vi "Redis@PreviewQueue__Parameter.vi"(1 "ParamterIn":string) -> (0 "ParamterOut":string)   [LabVIEW 2020]
panel:
  in  "Message=":string
  in  "TimeOut=":string(combo)
  in  "Variable=":string(combo)
  in  "Section":string(combo)
  in  "CMD":string
  in  "RedisSession":string(combo)
  in  "Confirm":bool
  # "RedisSession(,Variable=,TimeOut=XXX, Message=XXX)"
  # "@"
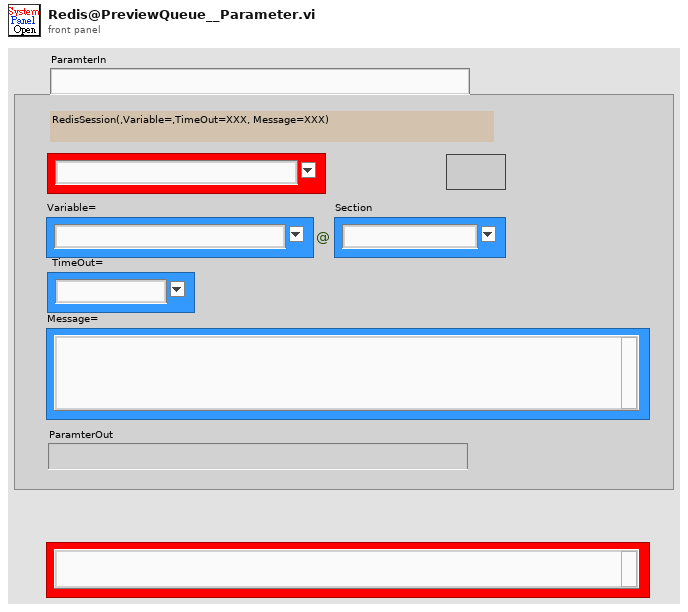
[diagram p1: front panel]
types:
  T1 = enum16{"Get", "Init", "Set", "Delete", "GetElement", "Inc", "Dec"}
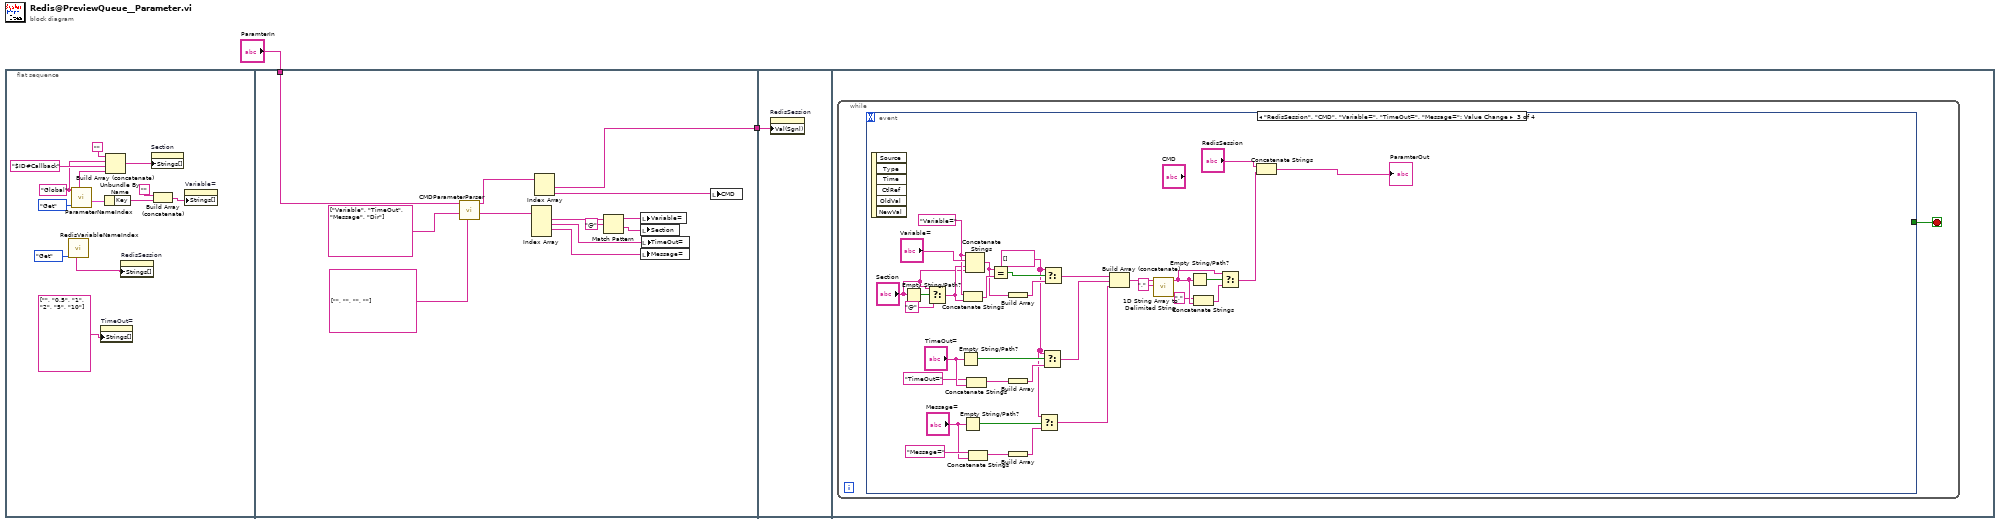
[diagram p0: block diagram]
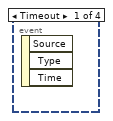
[diagram p2: hidden frame]
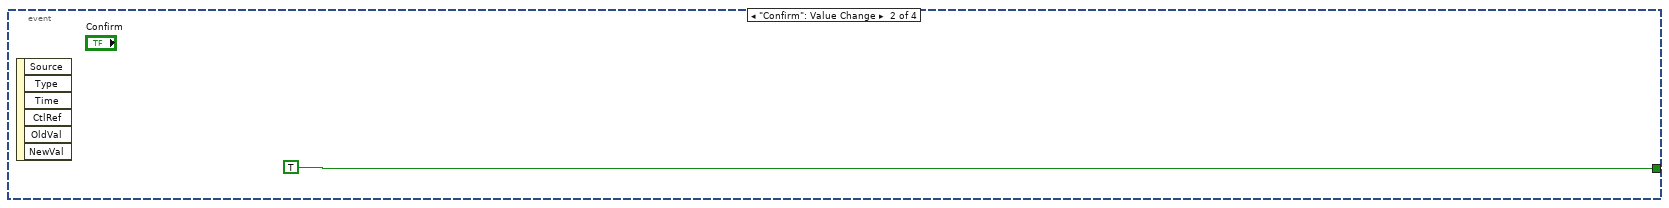
[diagram p3: hidden frame]
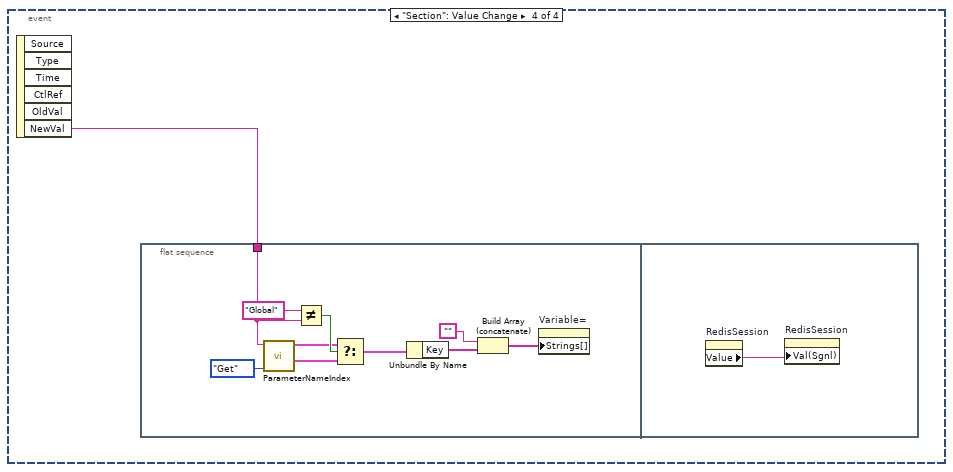
[diagram p4: hidden frame]
diagram:
  n1 = flat-sequence {
    tunnel: "ParamterIn" -> [w28]
    tunnel: [w24] -> w1
    tunnel: w1 -> [w29]
    frame #0 {
      w6 = "Global" ("VariableSection")
      n2 = call "RedisVariableNameIndex.vi"("OP"=enum16{"Add", "Init", "Get"}."Get") -> ("RedisSessionS"=w8:string[])  [unwired: 6 in, 4 out]
      n3 = call "ParameterNameIndex.vi"("OP"=T1."Get", "VariableSection"=w6) -> ("GlobalKeyValue"=w7:cluster{"Key":string[], "Value":string[]}, "SectionList"=w14:string[])  [unwired: 3 in, 5 out]
      n4 = property on="TimeOut=" class="CmbBox"("Strings[]"=string[] ["", "0.5", "1", "2", "5", "10"] ("Strings []")) -> ()  [unwired: 2 in, 2 out]
      n5 = Unbundle By Name(w7) -> ("Key"=w4:string[])
      n6 = Build Array (concatenate)("", w6, "$ID#Callback" ("VariableSection"), w14) -> (w13:string[])
      n7 = property on="RedisSession" class="CmbBox"("Strings[]"=w8) -> ()  [unwired: 2 in, 2 out]
      n8 = property on="Section" class="CmbBox"("Strings[]"=w13) -> ()  [unwired: 2 in, 2 out]
      n9 = Build Array (concatenate)("", w4) -> (w3:string[])
      n10 = property on="Variable=" class="CmbBox"("Strings[]"=w3) -> ()  [unwired: 2 in, 2 out]
    }
    frame #1 {
      n11 = call "CMDParameterParser.vi"("DeafultValues"=string[] ["", "", "", ""], "RequiredKeys"=string[] ["Variable", "TimeOut", "Message", "Dir"], "CMDParameter"=w28) -> ("KeyValues"=w22:string[], "Input"=w25:string[])  [unwired: 6 in, 1 out]
      n12 = Index Array(array=w22) -> (element #1=w21:string, element #2=w18:string, element #3=w17:string)  [unwired: 4 in, 1 out]
      n13 = Index Array(array=w25) -> (element #1=w24:string, element #2=w23:string)  [unwired: 2 in]
      n14 = Match Pattern(string=w21, regular expression="@") -> (before substring=w19:string, after substring=w16:string)  [unwired: 1 in, 2 out]
      n15 = local write "Variable="(w19) -> ()
      n16 = local write "Section"(w16) -> ()
      n17 = local write "Message="(w17) -> ()
      n18 = local write "TimeOut="(w18) -> ()
      n19 = local write "CMD"(w23) -> ()
    }
    frame #2 {
      n20 = property on="RedisSession" class="CmbBox"("Val(Sgnl)"=w29) -> ()  [unwired: 2 in, 2 out]
    }
    frame #3 {
      n21 = while {
        stop <- w30 stop-if-true
        n22 = event shown="[2] \"RedisSession\", \"CMD\", \"Variable=\", \"TimeOut=\", \"Message=\": Value Change" {
          selector: _ -> [_ _ _ _]
          dyn-events: _ -> [_ _ _ _]
          timeout: _ -> [_ _ _ _]
          tunnel: [_ TRUE _ _] -> w30
          event Timeout {
            n23 = event-data() -> ()  [unwired: 1 in, 3 out]
          }
          event "Confirm": Value Change {
            n24 = event-data() -> ()  [unwired: 1 in, 6 out]
          }
          event "RedisSession", "CMD", "Variable=", "TimeOut=", "Message=": Value Change {
            w47 = string[] [] ("t")
            w60 = "Variable=" ("string")
            n25 = event-data() -> ()  [unwired: 1 in, 6 out]
            n26 = Empty String/Path?(string/path="Section") -> (empty?=w36:bool)
            n27 = Select(t="Section", s=w36, f="@") -> (s? t:f=w34:string)
            n28 = Empty String/Path?(string/path="TimeOut=") -> (empty?=w59:bool)
            n29 = Empty String/Path?(string/path="Message=") -> (empty?=w54:bool)
            n30 = Concatenate Strings(w60, w34) -> (w53:string)
            n31 = Concatenate Strings(w60, "Variable=", w34, "Section") -> (w37:string)
            n32 = Concatenate Strings("TimeOut=" ("string"), "TimeOut=") -> (w51:string)
            n33 = Concatenate Strings("Message=" ("string"), "Message=") -> (w49:string)
            n34 = Equal?(x=w37, y=w53) -> (x = y?=w61:bool)
            n35 = Build Array(w37) -> (w52:string[])
            n36 = Build Array(w51) -> (w50:string[])
            n37 = Build Array(w49) -> (w48:string[])
            n38 = Select(t=w47, s=w54, f=w48) -> (s? t:f=w44:string[])
            n39 = Select(t=w47, s=w59, f=w50) -> (s? t:f=w45:string[])
            n40 = Select(t=w47, s=w61, f=w52) -> (s? t:f=w46:string[])
            n41 = Build Array (concatenate)(w46, w45, w44) -> (w43:string[])
            n42 = call <vilib>:"1D String Array to Delimited String.vi"("delimiter"=",", "string array"=w43) -> ("delimited string"=w40:string)  [unwired: 9 in]
            n43 = Empty String/Path?(string/path=w40) -> (empty?=w41:bool)
            n44 = Concatenate Strings("," ("string"), w40) -> (w38:string)
            n45 = Select(t=w40, s=w41, f=w38) -> (s? t:f=w32:string)
            n46 = Concatenate Strings("RedisSession", w32) -> (→"ParamterOut":string)
          }
          event "Section": Value Change {
            n47 = event-data() -> ("NewVal"=w65:string)  [unwired: 1 in, 5 out]
            n48 = flat-sequence {
              tunnel: w65 -> [w74]
              frame #0 {
                n49 = call "ParameterNameIndex.vi"("OP"=T1."Get", "VariableSection"=w74) -> ("GlobalKeyValue"=w70:cluster{"Key":string[], "Value":string[]}, "SectionKeyValue"=w71:cluster{"Key":string[], "Value":string[]})  [unwired: 3 in, 5 out]
                n50 = Not Equal?(x="Global", y=w74) -> (x != y?=w72:bool)
                n51 = Select(t=w71, s=w72, f=w70) -> (s? t:f=w69:cluster{"Key":string[], "Value":string[]})
                n52 = Unbundle By Name(w69) -> ("Key"=w68:string[])
                n53 = Build Array (concatenate)("", w68) -> (w66:string[])
                n54 = property on="Variable=" class="CmbBox"("Strings[]"=w66) -> ()  [unwired: 2 in, 2 out]
              }
              frame #1 {
                n55 = property on="RedisSession" class="CmbBox"() -> ("Value"=w76:string)  [unwired: 2 in, 2 out]
                n56 = property on="RedisSession" class="CmbBox"("Val(Sgnl)"=w76) -> ()  [unwired: 2 in, 2 out]
              }
            }
          }
        }
      }
    }
  }
